vi "Pre Launch Init.vi"(11 "DER in":refnum<class "DER.lvclass">) -> (0 "error out":errorcluster, 3 "DER out":refnum<class "DER.lvclass">)   [LabVIEW 2018, in "DER Actor.lvlib" / "DER.lvclass"]
doc: "(<B>Filename</B>: Actor Framework.lvlib:Actor.lvclass:Pre Launch Init.vi)\n\nDefines behavior that occurs after the Launch Nested Actor method is invoked but before the actor's Actor Core method begins running.\n\nBy default, this method does nothing. A descendant class may override it to define behavior."
uses:
  DER.lvclass
  C:/Users/Administrator/Desktop/2018LabVIEW EMS/EMS Generic Actor/EMS Generic/EMS Generic.lvclass
  C:/Users/Administrator/Desktop/2018LabVIEW EMS/IED Actors/Device DDS Communications Framework/Device DDS Communications/Device DDS Communications.lvclass
  Device DDS Communications Framework/Device DDS Communications/Device DDS Communications.lvclass/Device DDS Communications.ctl
  <vilib>/ORNL/CSEISMIC DDS/CSEISMIC DDS Base/CSEISMIC DDS.lvclass/CSEISMIC DDS.ctl
  <vilib>/ORNL/CSEISMIC DDS/CSEISMIC DDS Base/Accessors/Write DDS Reference.vi
  <vilib>/ORNL/CSEISMIC DDS/DDS Writer/DDS Writer.lvclass
  C:/Program Files (x86)/National Instruments/LabVIEW 2018/vi.lib/ORNL/CSEISMIC DDS/CSEISMIC DDS Base/CSEISMIC DDS.lvclass
  <vilib>/ORNL/CSEISMIC DDS/CSEISMIC DDS Base/Error Handler.vi
  Device DDS Communications Framework/Device DDS Communications/Device DDS Communications.lvclass
  EMS Generic Actor/EMS Generic/EMS Generic.lvclass
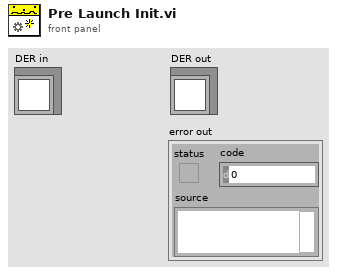
[diagram p1: front panel]
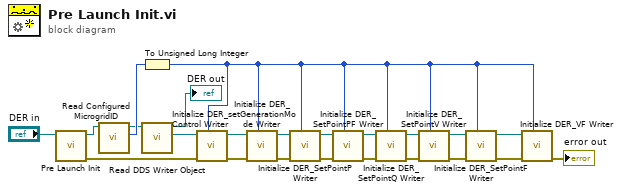
[diagram p0: block diagram]
diagram:
  n1 = call-parent "Pre Launch Init.vi"("Device DDS Communications in"="DER in") -> ("error out"=w6:errorcluster, "Device DDS Communications out"=w9:refnum<class "DER.lvclass">)  [unwired: 9 in]
  n2 = call "Read Configured MicrogridID.vi"("EMS Generic in"=w9) -> ("Microgrid ID"=w10:u8, "EMS Generic out"=w8:refnum<class "DER.lvclass">)  [unwired: 8 in, 1 out]
  n3 = To Unsigned Long Integer(number=w10) -> (unsigned 32bit integer=w1:u32)
  n4 = call "Read DDS Writer Object.vi"("Device DDS Communications in"=w8) -> ("DDS Writer Object"=w12:refnum<class "DDS Writer.lvclass">, "Device DDS Communications out"=→"DER out":refnum<class "DER.lvclass">)  [unwired: 9 in]
  n5 = call <vilib>:"Initialize DER_Control Writer.vi"("MicrogridID"=w1, "error in"=w6, "DDS Writer in"=w12) -> ("error out"=w23:errorcluster, "DDS Writer out"=w22:refnum<class "DDS Writer.lvclass">)  [unwired: 7 in]
  n6 = call <vilib>:"Initialize DER_setGenerationMode Writer.vi"("MicrogridID"=w1, "error in"=w23, "DDS Writer in"=w22) -> ("error out"=w21:errorcluster, "DDS Writer out"=w20:refnum<class "DDS Writer.lvclass">)  [unwired: 7 in]
  n7 = call <vilib>:"Initialize DER_SetPointP Writer.vi"("MicrogridID"=w1, "error in"=w21, "DDS Writer in"=w20) -> ("error out"=w19:errorcluster, "DDS Writer out"=w18:refnum<class "DDS Writer.lvclass">)  [unwired: 7 in]
  n8 = call <vilib>:"Initialize DER_SetPointPF Writer.vi"("MicrogridID"=w1, "error in"=w19, "DDS Writer in"=w18) -> ("error out"=w17:errorcluster, "DDS Writer out"=w16:refnum<class "DDS Writer.lvclass">)  [unwired: 7 in]
  n9 = call <vilib>:"Initialize DER_SetPointQ Writer.vi"("MicrogridID"=w1, "error in"=w17, "DDS Writer in"=w16) -> ("error out"=w15:errorcluster, "DDS Writer out"=w14:refnum<class "DDS Writer.lvclass">)  [unwired: 7 in]
  n10 = call <vilib>:"Initialize DER_SetPointV Writer.vi"("MicrogridID"=w1, "error in"=w15, "DDS Writer in"=w14) -> ("error out"=w5:errorcluster, "DDS Writer out"=w4:refnum<class "DDS Writer.lvclass">)  [unwired: 7 in]
  n11 = call <vilib>:"Initialize DER_SetPointF Writer.vi"("MicrogridID"=w1, "error in"=w5, "DDS Writer in"=w4) -> ("error out"=w2:errorcluster, "DDS Writer out"=w3:refnum<class "DDS Writer.lvclass">)  [unwired: 7 in]
  n12 = call <vilib>:"Initialize DER_VF Writer.vi"("MicrogridID"=w1, "error in"=w2, "DDS Writer in"=w3) -> ("error out"=→"error out":errorcluster)  [unwired: 7 in, 1 out]
